vi "deleteFile.vi"(8 "에러 입력":errorcluster, 9 "검색 문자열":string="시간", 10 "검색할 행수":i32=3, 11 "파일 경로":path) -> (0 "에러 출력":errorcluster, 3 "deleted":bool)   [LabVIEW 2018]
uses:
  <vilib>/Utility/file.llb/Read Delimited Spreadsheet (string).vi
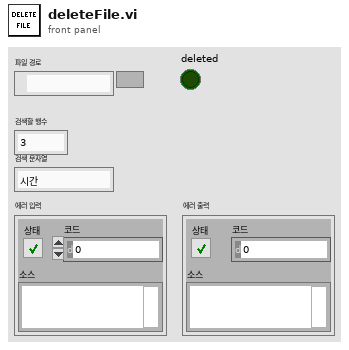
[diagram p1: front panel]
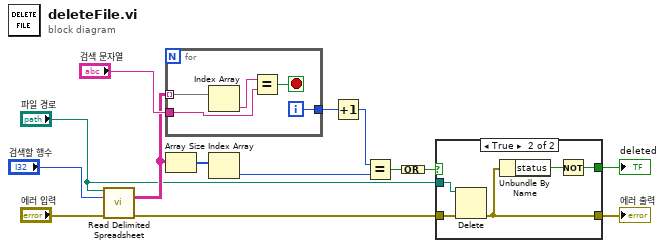
[diagram p0: block diagram]
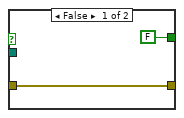
[diagram p2: hidden frame]
diagram:
  n1 = call-poly <vilib>:"Read Delimited Spreadsheet.vi"("file path (dialog if empty)"="파일 경로", "number of rows (all:-1)"="검색할 행수", "error in (no error)"="에러 입력") -> ("all rows"=w7:string[][], "error out"=w10:errorcluster)  [unwired: 7 in, 4 out]
  n2 = for {
    tunnel: w7 -> [w16] mode=indexing
    tunnel: "검색 문자열" -> [w19]
    tunnel: [w17] -> w6
    i -> [w17]
    stop <- w18 stop-if-true
    n3 = Index Array(array=w16) -> (element=w15:string)  [unwired: 1 in]
    n4 = Equal?(x=w15, y=w19) -> (x = y?=w18:bool)
  }
  n5 = Array Size(array=w7) -> (size(s)=w9:i32[])
  n6 = Index Array(array=w9) -> (element=w4:i32)  [unwired: 1 in]
  n7 = Increment(x=w6) -> (x+1=w5:i32)
  n8 = Equal?(x=w5, y=w4) -> (x = y?=w3:bool)
  n9 = Compound Arithmetic op=OR ("복합 연산")(w3) -> (w8:bool)
  n10 = case shown="True" w8 {
    tunnel: "파일 경로" -> [_ w25]
    tunnel: w10 -> [w21 w26]
    tunnel: [w21 w24] -> w14
    tunnel: [FALSE w22] -> w1
    frame False {
    }
    frame True {
      n11 = Delete(path (use dialog)=w25, error in=w26) -> (error out=w24:errorcluster)  [unwired: 3 in, 2 out]
      n12 = Unbundle By Name(w24) -> ("status"=w23:bool)
      n13 = Not(x=w23) -> (.not. x?=w22:bool)
    }
  }
  "에러 출력" <- w14
  "deleted" <- w1
